vi "writeXML.vi"(8 "error in (no error)":errorcluster, 10 "Path":path, 11 "WinX32Settings in":refnum<class "WinX32Settings.lvclass">) -> (0 "error out":errorcluster, 3 "WinX32Settings out":refnum<class "WinX32Settings.lvclass">)   [LabVIEW 2011, in "Tools.lvlib" / "Settings.lvlib" / "WinX32Settings.lvclass"]
uses:
  WinX32Settings.lvclass
  NativeXML/NativeXML.lvclass
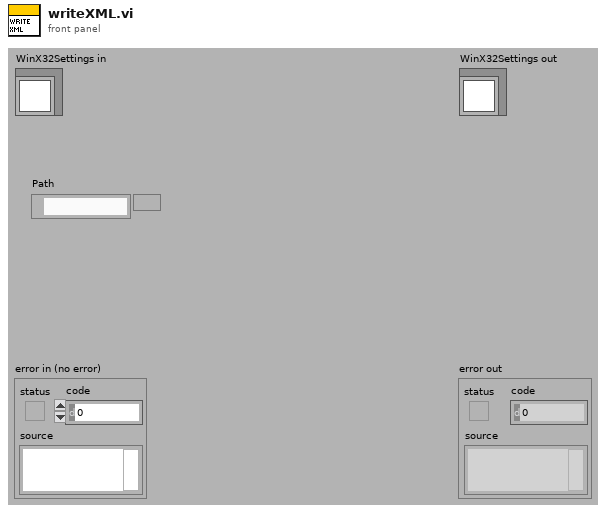
[diagram p1: front panel]
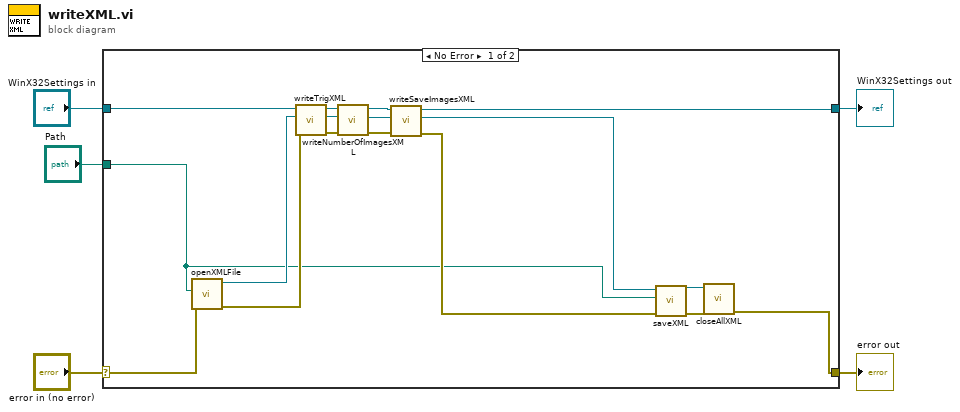
[diagram p0: block diagram]
diagram:
  n1 = case shown="No Error" "error in (no error)" {
    selector: "error in (no error)" -> [w20 w24]
    tunnel: [w6 w24] -> w4
    tunnel: [w10 w23] -> w2
    tunnel: "WinX32Settings in" -> [w18 w23]
    tunnel: "Path" -> [w7 _]
    frame No Error {
      n2 = call "openXMLFile.vi"("error in (no error)"=w20, "Path"=w7) -> ("error out"=w17:errorcluster, "NativeXML out"=w19:refnum<class "NativeXML.lvclass">)  [unwired: 8 in]
      n3 = call "writeTrigXML.vi"("error in (no error)"=w17, "NativeXML in"=w19, "WinX32Settings in"=w18) -> ("error out"=w14:errorcluster, "NativeXML out"=w15:refnum<class "NativeXML.lvclass">, "WinX32Settings out"=w16:refnum<class "WinX32Settings.lvclass">)  [unwired: 6 in]
      n4 = call "writeNumberOfImagesXML.vi"("error in (no error)"=w14, "NativeXML in"=w15, "WinX32Settings in"=w16) -> ("error out"=w11:errorcluster, "NativeXML out"=w12:refnum<class "NativeXML.lvclass">, "WinX32Settings out"=w13:refnum<class "WinX32Settings.lvclass">)  [unwired: 6 in]
      n5 = call "writeSaveImagesXML.vi"("error in (no error)"=w11, "NativeXML in"=w12, "WinX32Settings in"=w13) -> ("error out"=w9:errorcluster, "NativeXML out"=w8:refnum<class "NativeXML.lvclass">, "WinX32Settings out"=w10:refnum<class "WinX32Settings.lvclass">)  [unwired: 6 in]
      n6 = call "saveXML.vi"("error in (no error)"=w9, "Path"=w7, "NativeXML in"=w8) -> ("error out"=w22:errorcluster, "NativeXML out"=w21:refnum<class "NativeXML.lvclass">)  [unwired: 7 in]
      n7 = call "closeAllXML.vi"("error in (no error)"=w22, "NativeXML in"=w21) -> ("error out"=w6:errorcluster)  [unwired: 9 in]
    }
    frame Error {
    }
  }
  "error out" <- w4
  "WinX32Settings out" <- w2
